vi "getState.vi"(8 "error in (no error)":errorcluster, 11 "ISA010 in":refnum<class "ISA010.lvclass">) -> (0 "error out":errorcluster, 2 "ISA010State":string, 3 "ISA010 out":refnum<class "ISA010.lvclass">)   [LabVIEW 2015, in "ISA010.lvlib" / "ISA010.lvclass"]
uses:
  ISA010.lvclass
  libraries/ModBUS.lvlibp/ASCII/ASCII.lvclass
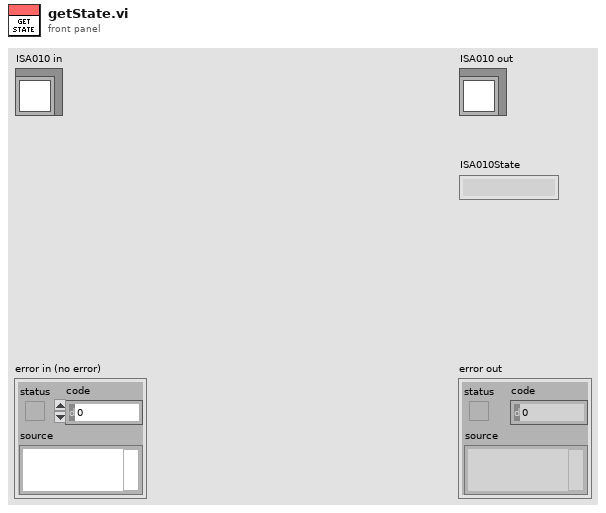
[diagram p1: front panel]
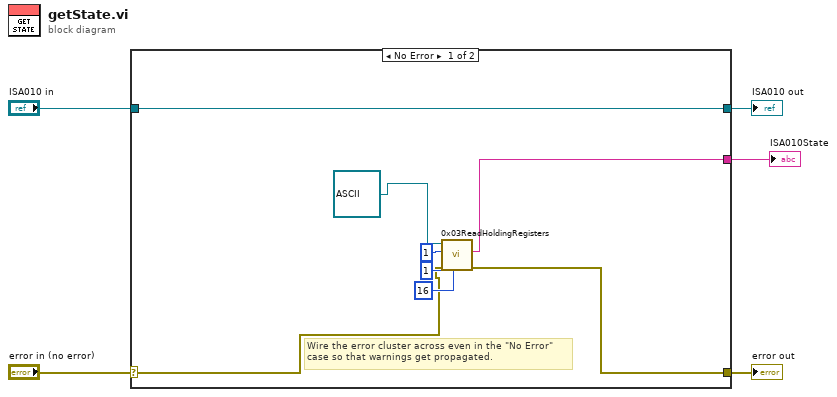
[diagram p0: block diagram]
diagram:
  n1 = case shown="No Error" "error in (no error)" {
    selector: "error in (no error)" -> [w9 w15]
    tunnel: [w8 w15] -> w4
    tunnel: [w13 w14] -> w2
    tunnel: "ISA010 in" -> [w13 w14]
    tunnel: [w7 _] -> w1
    frame No Error {
      # "Wire the error cluster across even in the \"No Error\"\ncase so that warnings get propagated."
      n2 = call-dynamic "0x03ReadHoldingRegisters.vi"("Length 2"=u16 16, "error in (no error)"=w9, "Register"=u16 1, "Addressc"=u8 1, "ASCII in"=refnum<class "ASCII.lvclass"> refnum ("ModBUS.lvlibp:ASCII.lvclass")) -> ("error out"=w8:errorcluster, "Frame"=w7:string)  [unwired: 4 in, 1 out]
    }
    frame Error {
    }
  }
  "error out" <- w4
  "ISA010 out" <- w2
  "ISA010State" <- w1
